vi "Actor Core.vi"(8 "error in":errorcluster, 11 "Nested in":refnum<class "Generador funciones.lvclass">) -> (0 "error out":errorcluster, 3 "Actor out":refnum<class "Actor.lvclass">)   [LabVIEW 2019, in "Generador funciones.lvlib" / "Generador funciones.lvclass"]
doc: "(<B>Filename</B>: Actor Framework.lvlib:Actor.lvclass:Actor Core.vi)\n\nReceives messages to the actor, reacts to them, and initiates any error handling that may shut the actor down.\n\nDescendant classes may override this VI to append parallel tasks for the actor to complete while it handles messages. Overrides use the Call Parent Method node."
uses:
  Generador funciones.lvclass
  C:/Program Files/National Instruments/LabVIEW 2019/vi.lib/ActorFramework/Actor/Actor.lvclass
  <vilib>/ActorFramework/Actor/Actor.lvclass
  Generador funciones ACQ/Generador funciones ACQ.lvclass
  Generador funciones.lvclass/Generador funciones.ctl
  <vilib>/ActorFramework/Actor/Actor.lvclass/Actor.ctl
  <vilib>/ActorFramework/Message Enqueuer/Message Enqueuer.lvclass/Message Enqueuer.ctl
  Generador funciones Messages/StartStop Msg/StartStop Msg.lvclass/StartStop Msg.ctl
  Generador funciones Messages/Amplitud Msg/Amplitud Msg.lvclass/Amplitud Msg.ctl
  Generador funciones Messages/Frecuencia Msg/Frecuencia Msg.lvclass/Frecuencia Msg.ctl
  <vilib>/ActorFramework/Message Enqueuer/Init from Existing Queue.vi
  <vilib>/ActorFramework/Message Enqueuer/Enqueue.vi
  <vilib>/Utility/error.llb/Clear Errors.vi
  <vilib>/ActorFramework/Stop Msg/Stop Msg.lvclass
  C:/Program Files/National Instruments/LabVIEW 2019/vi.lib/ActorFramework/Message/Message.lvclass
  Generador funciones Messages/StartStop Msg/StartStop Msg.lvclass
  Generador funciones Messages/Amplitud Msg/Amplitud Msg.lvclass
  Generador funciones Messages/Frecuencia Msg/Frecuencia Msg.lvclass
  <vilib>/ActorFramework/Message Priority Queue/Priority Enqueue.vi
  <vilib>/ActorFramework/Message Enqueuer/Message Enqueuer.lvclass
panel:
  out "Graph":waveform(dbl)(graph)
  out "Grafica":dbl(graph)
  in  "Tipo de Señal":u16(ring) items=["please select", "Senoidal", "Triangular", "Cuadrada"]
  in  "Frecuencia":dbl
  in  "Amplitud":dbl
  in  "Save":bool
  in  "Format":enum16{"select", "txt", "tdms"}(ring)
  in  "Path":path
  in  "Stop":bool
  in  "Start":bool
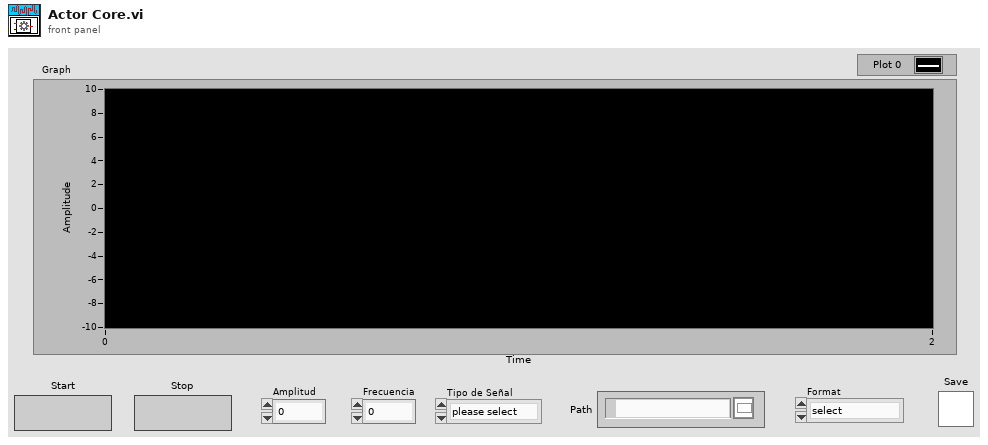
[diagram p1: front panel]
types:
  T1 = cluster{"Stop":refnum<user-event>, "Grafica":refnum<user-event>, "Graph":refnum<user-event>}
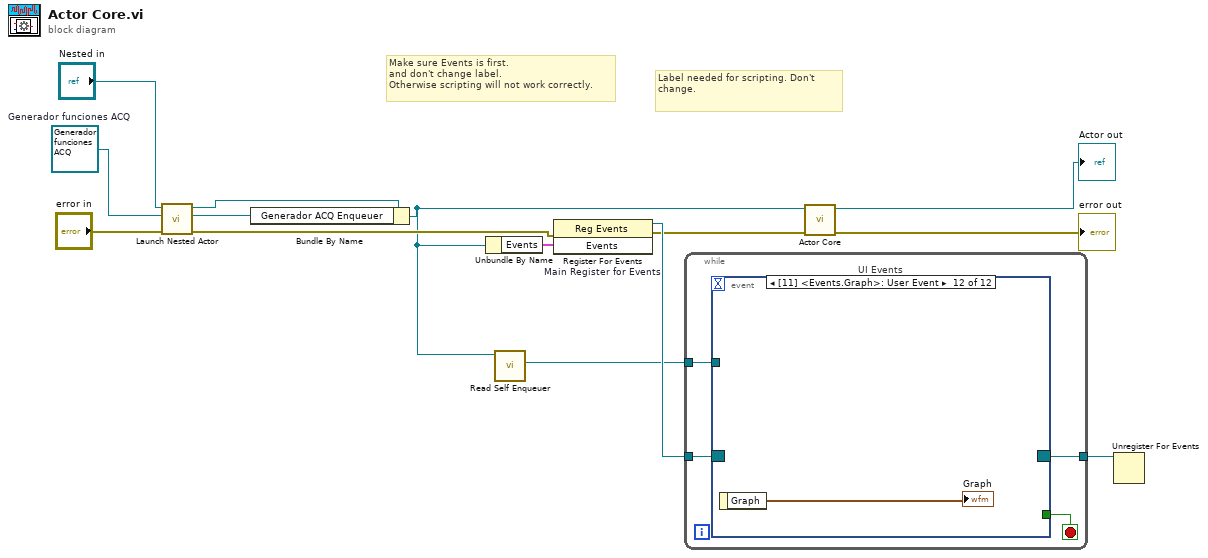
[diagram p0: block diagram]
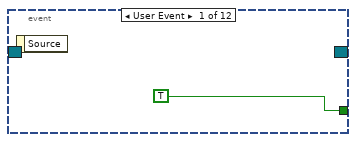
[diagram p2: hidden frame]
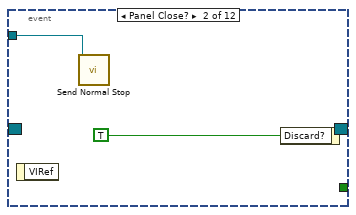
[diagram p3: hidden frame]
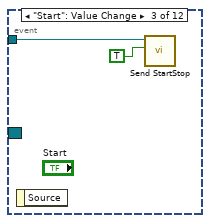
[diagram p4: hidden frame]
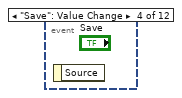
[diagram p5: hidden frame]
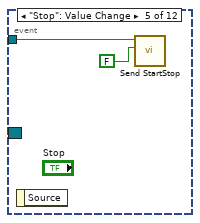
[diagram p6: hidden frame]
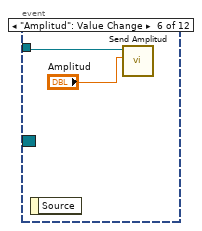
[diagram p7: hidden frame]
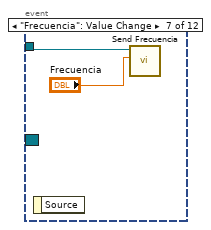
[diagram p8: hidden frame]
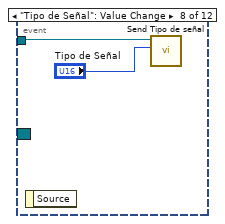
[diagram p9: hidden frame]
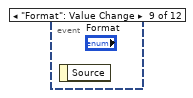
[diagram p10: hidden frame]
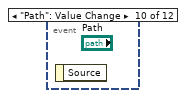
[diagram p11: hidden frame]
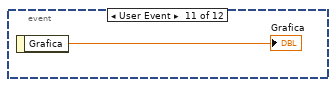
[diagram p12: hidden frame]
diagram:
  w4 = refnum<class "Generador funciones ACQ.lvclass"> refnum  # Generador funciones ACQ
  # "Label needed for scripting. Don't change."
  # "Make sure Events is first.\nand don't change label.\nOtherwise scripting will not work correctly."
  n1 = call <vilib>:"Launch Nested Actor.vi"("error in (no error)"="error in", "Nested Actor"=w4, "Caller Actor in"="Nested in") -> ("error out"=w6:errorcluster, "Nested Actor's Enqueuer"=w2:refnum<class "Message Enqueuer.lvclass">, "Caller Actor out"=w3:refnum<class "Generador funciones.lvclass">)  [unwired: 6 in]
  n2 = Bundle By Name(cluster=w3, "Generador ACQ Enqueuer"=w2) -> (w1:refnum<class "Generador funciones.lvclass">)
  n3 = Unbundle By Name(w1) -> ("Events"=w11:T1)
  n4 = call <vilib>:"Read Self Enqueuer.vi"("Actor"=w1) -> ("Self Enqueuer"=w9:refnum<class "Message Enqueuer.lvclass">)  [unwired: 10 in]
  n5 = register-events "Main Register for Events"(error in=w6, w11) -> (reference out=w12:refnum<event-registration>, error out=w8:errorcluster)  [unwired: 1 in]
  n6 = while {
    tunnel: w12 -> [w18]
    tunnel: [w16] -> w10
    tunnel: w9 -> [w15]
    stop <- w17 stop-if-true
    n7 = event "UI Events" shown="[11] <Events.Graph>: User Event" {
      selector: w18 -> [_ _ _ _ _ _ _ _ _ _ _ _]
      dyn-events: [_ _ _ _ _ _ _ _ _ _ _ _] -> w16
      timeout: _ -> [_ _ _ _ _ _ _ _ _ _ _ _]
      tunnel: [TRUE _ _ _ _ _ _ _ _ _ _ _] -> w17
      tunnel: w15 -> [_ w20 w23 _ w25 w27 w29 w31 _ _ _ _]
      event User Event {
        n8 = event-data() -> ()  [unwired: 1 in, 1 out]
      }
      event Panel Close? {
        n9 = event-data() -> ()  [unwired: 1 in, 1 out]
        n10 = call <vilib>:"Send Normal Stop.vi"("Message Enqueuer"=w20) -> ()  [unwired: 10 in, 1 out]
        n11 = event-data("Discard?"=TRUE) -> ()  [unwired: 1 in, 1 out]
      }
      event "Start": Value Change {
        n12 = event-data() -> ()  [unwired: 1 in, 1 out]
        n13 = call "Send StartStop.vi"("Start/Stop"=TRUE, "Message Enqueuer"=w23) -> ()  [unwired: 8 in, 2 out]
      }
      event "Save": Value Change {
        n14 = event-data() -> ()  [unwired: 1 in, 1 out]
      }
      event "Stop": Value Change {
        n15 = event-data() -> ()  [unwired: 1 in, 1 out]
        n16 = call "Send StartStop.vi"("Start/Stop"=FALSE, "Message Enqueuer"=w25) -> ()  [unwired: 8 in, 2 out]
      }
      event "Amplitud": Value Change {
        n17 = event-data() -> ()  [unwired: 1 in, 1 out]
        n18 = call "Send Amplitud.vi"("Amplitud"="Amplitud", "Message Enqueuer"=w27) -> ()  [unwired: 8 in, 2 out]
      }
      event "Frecuencia": Value Change {
        n19 = event-data() -> ()  [unwired: 1 in, 1 out]
        n20 = call "Send Frecuencia.vi"("Frecuencia"="Frecuencia", "Message Enqueuer"=w29) -> ()  [unwired: 8 in, 2 out]
      }
      event "Tipo de Señal": Value Change {
        n21 = event-data() -> ()  [unwired: 1 in, 1 out]
        n22 = call "Send Tipo de señal.vi"("Tipo de señal"="Tipo de Señal", "Message Enqueuer"=w31) -> ()  [unwired: 8 in, 2 out]
      }
      event "Format": Value Change {
        n23 = event-data() -> ()  [unwired: 1 in, 1 out]
      }
      event "Path": Value Change {
        n24 = event-data() -> ()  [unwired: 1 in, 1 out]
      }
      event User Event {
        n25 = event-data() -> ("Grafica"=→"Grafica":dbl)  [unwired: 1 in]
      }
      event User Event {
        n26 = event-data() -> ("Graph"=→"Graph":waveform(dbl))  [unwired: 1 in]
      }
    }
  }
  n27 = call-parent "Actor Core.vi"("error in"=w8, "Actor in"=w1) -> ("error out"=→"error out":errorcluster, "Actor out"=→"Actor out":refnum<class "Actor.lvclass">)  [unwired: 8 in]
  n28 = Unregister For Events(event registration refnum=w10) -> ()  [unwired: 1 in, 1 out]
